vi "Read Buffered Error.vi"(7 "Reset":bool, 8 "error in":errorcluster, 9 "timeout in ms (0)":i32, 11 "Engine Runtime Interface in":refnum<class "Engine Runtime Interface.lvclass">) -> (0 "error out":errorcluster, 2 "Engine Error":errorcluster, 3 "Engine Runtime Interface out":refnum<class "Engine Runtime Interface.lvclass">)   [LabVIEW 2014, in "Engine Runtime Interface.lvclass"]
doc: "Reads any critical engine errors that may have occurred. For recoverable module problems, use Read Fault List.vi"
uses:
  Engine Runtime Interface.lvclass
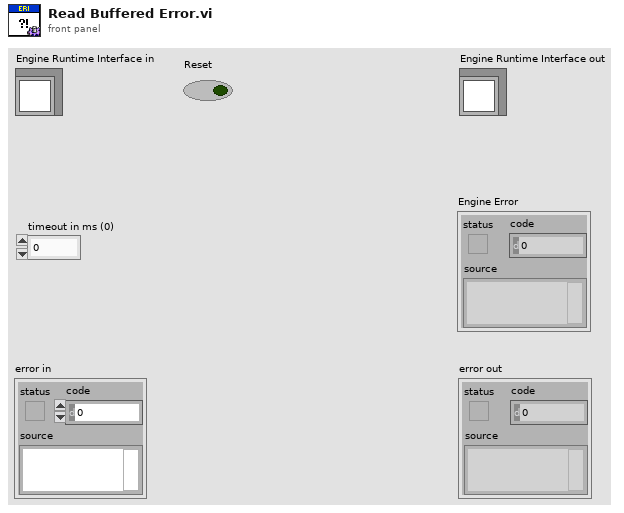
[diagram p1: front panel]
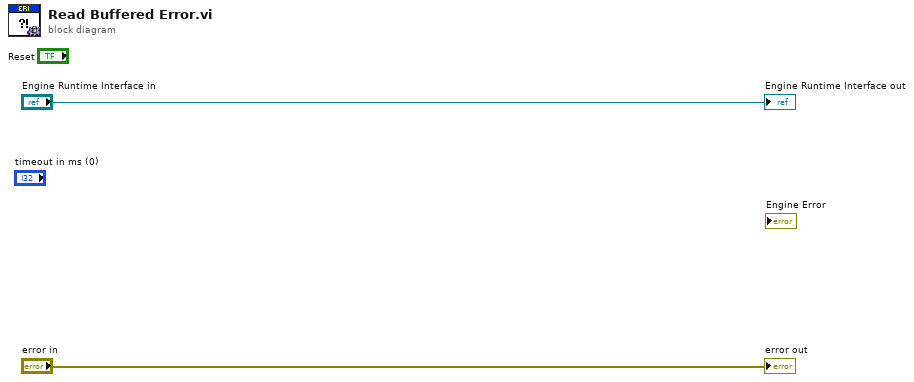
[diagram p0: block diagram]
diagram:
  "error out" <- "error in"
  "Engine Runtime Interface out" <- "Engine Runtime Interface in"
